vi "Comparar precios Coca.vi"(6 "Inventario":string, 8 "error in (no error)":errorcluster, 9 "Precio":string, 10 "Producto":string, 11 "UI Actor in":refnum<class "UI Actor.lvclass">) -> (0 "error out":errorcluster, 3 "UI Actor out":refnum<class "UI Actor.lvclass">)   [LabVIEW 2020, in "UI Actor.lvlib" / "UI Actor.lvclass"]
uses:
  UI Actor.lvclass
  UI Actor.lvclass/UI Actor.ctl
  Msg Messages/Update Msg Msg/Update Msg Msg.lvclass/Update Msg Msg.ctl
  <vilib>/ActorFramework/Message Enqueuer/Message Enqueuer.lvclass/Message Enqueuer.ctl
  Coca Actor Messages/Act Inventario Msg/Act Inventario Msg.lvclass/Act Inventario Msg.ctl
  <vilib>/ActorFramework/Message Enqueuer/Enqueue.vi
  Msg Messages/Update Msg Msg/Update Msg Msg.lvclass
  C:/Program Files (x86)/National Instruments/LabVIEW 2020/vi.lib/ActorFramework/Message/Message.lvclass
  Coca Actor Messages/Act Inventario Msg/Act Inventario Msg.lvclass
  Coca Actor Messages/Act Tabla Msg/Act Tabla Msg.lvclass
  <vilib>/ActorFramework/Message Priority Queue/Priority Enqueue.vi
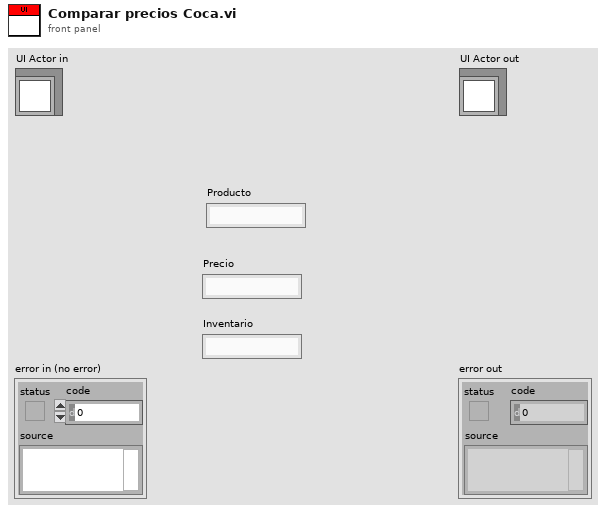
[diagram p1: front panel]
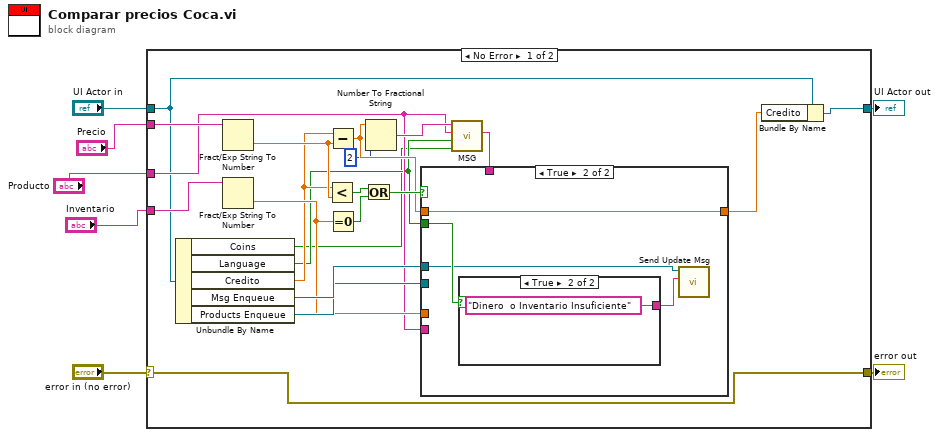
[diagram p0: block diagram]
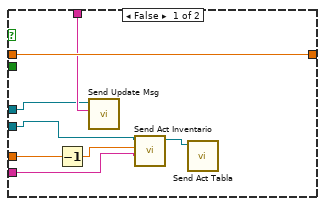
[diagram p2: hidden frame]
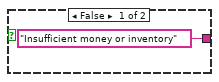
[diagram p3: hidden frame]
diagram:
  n1 = case shown="No Error" "error in (no error)" {
    selector: "error in (no error)" -> [w10 w44]
    tunnel: [w10 w44] -> w6
    tunnel: [w11 w43] -> w4
    tunnel: "UI Actor in" -> [w12 w43]
    tunnel: "Precio" -> [w16 _]
    tunnel: "Inventario" -> [w15 _]
    tunnel: "Producto" -> [w14 _]
    frame No Error {
      n2 = Unbundle By Name(w12) -> ("Coins"=w8:bool, "Language"=w9:bool, "Credito"=w13:dbl, "Msg Enqueue"=w28:refnum<class "Message Enqueuer.lvclass">, "Products Enqueue"=w27:refnum<class "Message Enqueuer.lvclass">)
      n3 = Fract/Exp String To Number(string=w16) -> (number=w21:dbl)  [unwired: 3 in, 1 out]
      n4 = Fract/Exp String To Number(string=w15) -> (number=w23:dbl)  [unwired: 3 in, 1 out]
      n5 = Less?(x=w13, y=w21) -> (x < y?=w25:bool)
      n6 = Subtract(x=w13, y=w21) -> (x-y=w22:dbl)
      n7 = Equal To 0?(x=w23) -> (x = 0?=w24:bool)
      n8 = Or(x=w25, y=w24) -> (x .or. y?=w26:bool)
      n9 = Number To Fractional String(number=w22, precision (6)=i16 2) -> (F-format string=w19:string)  [unwired: 2 in]
      n10 = call "MSG.vi"("Coins"=w8, "Language"=w9, "Producto"=w14, "String"=w19) -> ("concatenated string"=w18:string)  [unwired: 7 in]
      n11 = case shown="True" w26 {
        tunnel: w23 -> [w36 _]
        tunnel: w28 -> [w33 w37]
        tunnel: w27 -> [w30 _]
        tunnel: w9 -> [_ w38]
        tunnel: w22 -> [w35 w39]
        tunnel: [w35 w39] -> w20
        tunnel: w18 -> [w34 _]
        tunnel: w14 -> [w32 _]
        frame False {
          n12 = Decrement(x=w36) -> (x-1=w31:dbl)
          n13 = call "Send Update Msg.vi"("Update Msg"=w34, "Message Enqueuer"=w33) -> ()  [unwired: 8 in, 2 out]
          n14 = call "Send Act Inventario.vi"("Producto"=w32, "Inventario"=w31, "Message Enqueuer"=w30) -> ("Message Enqueuer out"=w29:refnum<class "Message Enqueuer.lvclass">)  [unwired: 7 in, 1 out]
          n15 = call "Send Act Tabla.vi"("Message Enqueuer"=w29) -> ()  [unwired: 9 in, 2 out]
        }
        frame True {
          n16 = case shown="True" w38 {
            tunnel: ["Insufficient money or inventory" ("Update Msg") "Dinero  o Inventario Insuficiente" ("Update Msg")] -> w40
            frame False {
            }
            frame True {
            }
          }
          n17 = call "Send Update Msg.vi"("Update Msg"=w40, "Message Enqueuer"=w37) -> ()  [unwired: 8 in, 2 out]
        }
      }
      n18 = Bundle By Name(cluster=w12, "Credito"=w20) -> (w11:refnum<class "UI Actor.lvclass">)
    }
    frame Error {
    }
  }
  "error out" <- w6
  "UI Actor out" <- w4
